vi "Create Node.vi"(7 "Node ID":u32, 8 "error in (no error)":errorcluster, 9 "Event Log Folder":path, 10 "Node Name":string, 11 "Cluster in":refnum<class "Cluster.lvclass">) -> (0 "error out":errorcluster, 2 "Node":refnum<class "Node.lvclass">, 3 "Cluster out":refnum<class "Cluster.lvclass">)   [LabVIEW 2020, in "VolatusConfig.lvlib" / "Cluster.lvclass"]
uses:
  Cluster.lvclass
  C:/dev/lv20CE/relink/lv-volatus/VolatusConfig/VolatusConfigElement/VolatusConfigElement.lvclass
  Node/Node.lvclass
  VolatusConfigElement/VolatusConfigElement.lvclass/VolatusConfigElement.ctl
  VolatusConfigElement/Element.vi
  VolatusConfigElement/VolatusConfigElement.lvclass
  lv-cdm/CDM-Config/Config Element/Config Element.lvclass
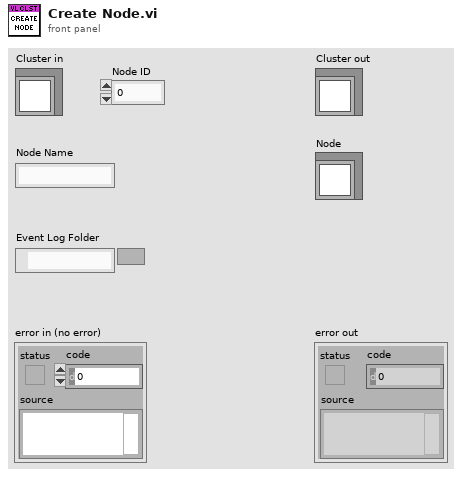
[diagram p1: front panel]
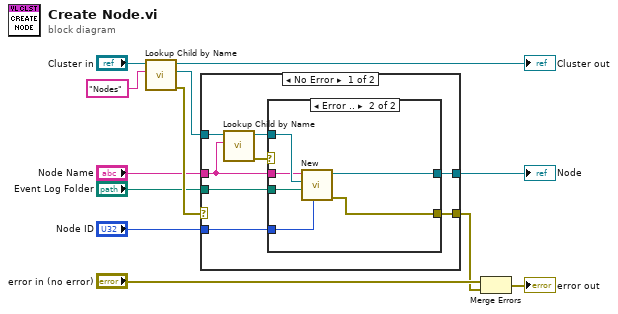
[diagram p0: block diagram]
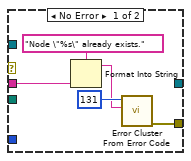
[diagram p2: hidden frame]
diagram:
  n1 = call "Lookup Child by Name.vi"("Child Name"="Nodes", "VolatusConfigElement in"="Cluster in") -> ("error out"=w7:errorcluster, "Child"=w8:refnum<class "Config Element.lvclass">, "VolatusConfigElement out"=→"Cluster out":refnum<class "Cluster.lvclass">)  [unwired: 6 in, 1 out]
  n2 = case shown="No Error" w7 {
    selector: w7 -> [_ w32]
    tunnel: w8 -> [w20 _]
    tunnel: "Node Name" -> [w17 _]
    tunnel: [w16 w32] -> w3
    tunnel: [w15 _] -> w5
    tunnel: "Event Log Folder" -> [w14 _]
    tunnel: "Node ID" -> [w13 _]
    frame No Error {
      n3 = call "Lookup Child by Name.vi"("Name"=w17, "Config Element in"=w20) -> ("error out"=w18:errorcluster, "Config Element out"=w19:refnum<class "Config Element.lvclass">)  [unwired: 6 in, 2 out]
      n4 = case shown="Error .." w18 {
        tunnel: w19 -> [_ w31]
        tunnel: w17 -> [w24 w30]
        tunnel: [w21 w29] -> w16
        tunnel: [_ w28] -> w15
        tunnel: w14 -> [_ w27]
        tunnel: w13 -> [_ w26]
        frame No Error {
          n5 = Format Into String(format string="Node \"%s\" already exists.", w24) -> (resulting string=w22:string)  [unwired: 2 in, 1 out]
          n6 = call <vilib>:"Error Cluster From Error Code.vi"("error message (\"\")"=w22, "error code (0)"=131) -> ("error out"=w21:errorcluster)  [unwired: 7 in]
        }
        frame Error {
          n7 = call "New.vi"("Node ID"=w26, "Event Log Folder"=w27, "Parent"=w31, "Name"=w30) -> ("error out"=w29:errorcluster, "Node out"=w28:refnum<class "Node.lvclass">)  [unwired: 6 in]
        }
      }
    }
    frame Error {
    }
  }
  "Node" <- w5
  n8 = Merge Errors("error in (no error)", w3) -> (→"error out":errorcluster)
